vi "julian date.vi"(10 "Day of the year":dbl, 11 "Year":dbl) -> (2 "Julian date of the day":dbl, 3 "Julian date of the year":dbl)   [LabVIEW 2015]
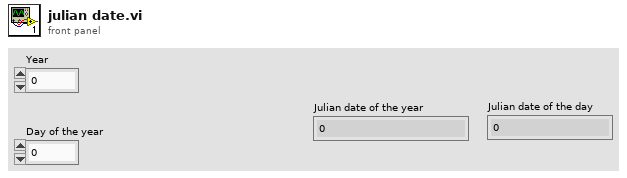
[diagram p1: front panel]
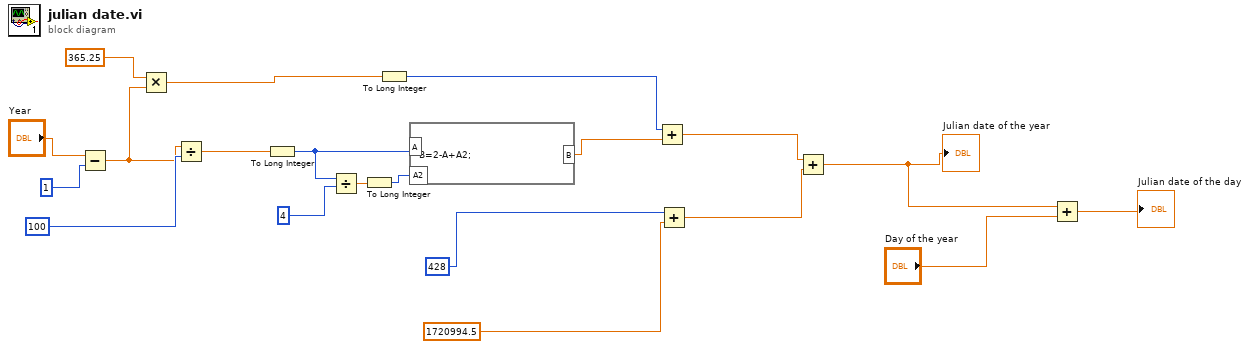
[diagram p0: block diagram]
diagram:
  n1 = Subtract(x="Year", y=1) -> (x-y=w12:dbl)
  n2 = Multiply(x=365.25, y=w12) -> (x*y=w10:dbl)
  n3 = Divide(x=w12, y=100) -> (x/y=w19:dbl)
  n4 = To Long Integer(number=w19) -> (32bit integer=w18:i32)
  n5 = Divide(x=w18, y=4) -> (x/y=w16:dbl)
  n6 = To Long Integer(number=w16) -> (32bit integer=w15:i32)
  n7 = To Long Integer(number=w10) -> (32bit integer=w9:i32)
  n8 = formula code="B=2-A+A2;"("A"=w18, "A2"=w15) -> ("B"=w8:dbl)
  n9 = Add(x=w9, y=w8) -> (x+y=w5:dbl)
  n10 = Add(x=428, y=1720994.5) -> (x+y=w4:dbl)
  n11 = Add(x=w5, y=w4) -> (x+y=w2:dbl)
  "Julian date of the year" <- w2
  n12 = Add(x=w2, y="Day of the year") -> (x+y=→"Julian date of the day":dbl)
